vi "TPulse.vi"(5 "input":bool, 7 "TPulse":i32, 11 "error in":errorcluster) -> (8 "output":bool, 15 "error out":errorcluster)   [LabVIEW 2022 SP3, in "BinarySignalProcessClass.lvclass"]
uses:
  BinarySignalProcessClass.lvclass
  <vilib>/functionblocks/FB Core/FB Core.xnode
  BinarySignalProcessClass.lvclass/BinarySignalProcessClass.ctl
  <vilib>/functionblocks/Counter/Pulse Timer/Pulse Timer.vi
  <vilib>/functionblocks/NI_FunctionBlock Libraries.lvlib
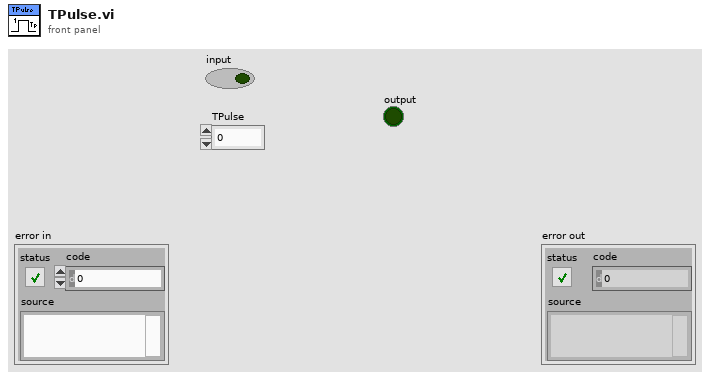
[diagram p1: front panel]
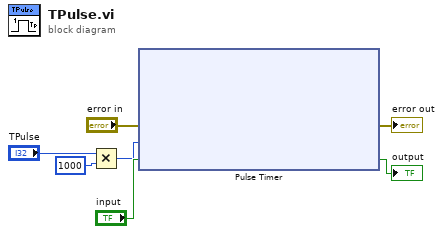
[diagram p0: block diagram]
diagram:
  n1 = Multiply(x="TPulse", y=1000) -> (x*y=w3:i32)
  n2 = xnode "Pulse Timer"("error in"="error in", "preset time (ms)"=w3, "input"="input") -> ("error out"=→"error out":errorcluster, "output"=→"output":bool)  [unwired: 1 out]
